vi "GetParameter.vi"(8 "error in (no error)":errorcluster, 10 "ID":u16, 11 "ZWO_ASI in":refnum<class "ZWO_ASI.lvclass">) -> (0 "error out":errorcluster, 2 "Value":string, 3 "ZWO_ASI out":refnum<class "ZWO_ASI.lvclass">)   [LabVIEW 2023, in "ZWO_ASI.lvlib" / "ZWO_ASI.lvclass"]
uses:
  ZWO_ASI.lvclass
  ZWO_ASI.lvclass/ZWO_ASI.ctl
  <userlib>/ASICamera2_no_err/ASICamera2_no_err.lvlib
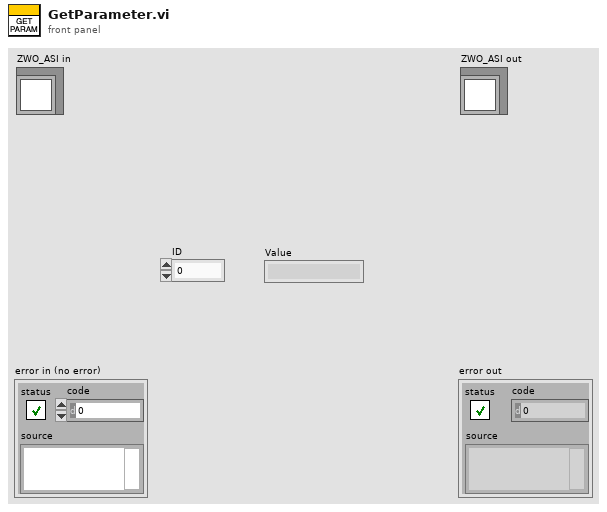
[diagram p1: front panel]
types:
  T1 = cluster{"name":string, "ControlType":u32, "plValue out":i32, "MaxValue":i32, "MinValue":i32}[]
  T2 = cluster{"name":string, "ControlType":u32, "plValue out":i32, "MaxValue":i32, "MinValue":i32}
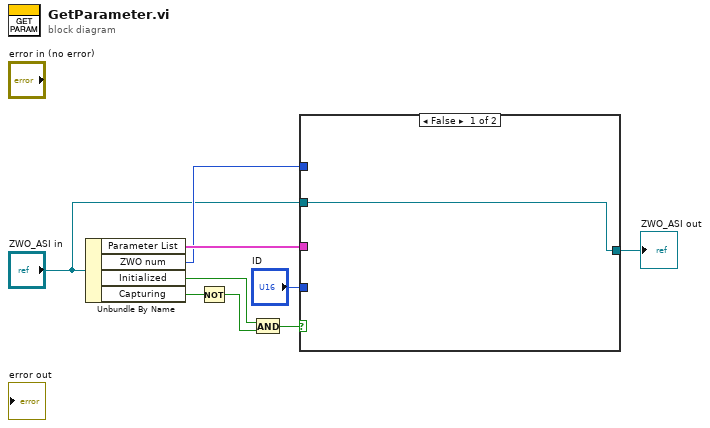
[diagram p0: block diagram]
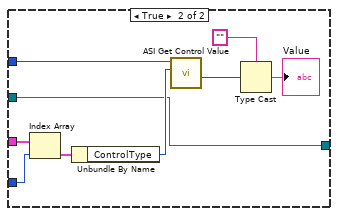
[diagram p2: hidden frame]
diagram:
  n1 = Unbundle By Name("ZWO_ASI in") -> ("Parameter List"=w9:T1, "ZWO num"=w7:i32, "Initialized"=w5:bool, "Capturing"=w4:bool)
  n2 = Not(x=w4) -> (.not. x?=w6:bool)
  n3 = And(x=w5, y=w6) -> (x .and. y?=w3:bool)
  n4 = case shown="False" w3 {
    tunnel: w9 -> [_ w19]
    tunnel: "ID" -> [_ w18]
    tunnel: w7 -> [_ w12]
    tunnel: [w10 w11] -> w2
    tunnel: "ZWO_ASI in" -> [w10 w11]
    frame False {
    }
    frame True {
      n5 = Index Array(array=w19, index=w18) -> (element=w17:T2)
      n6 = Unbundle By Name(w17) -> ("ControlType"=w14:u32)
      n7 = call <userlib>:"ASI Get Control Value.vi"("ControlType"=w14, "iCameraID"=w12) -> ("plValue out"=w13:i32)  [unwired: 7 in, 2 out]
      n8 = Type Cast(type="", x=w13) -> (*(type *) &x=→"Value":string)
    }
  }
  "ZWO_ASI out" <- w2
